vi "AudioStreamer.Close.vi"() -> (0 "success":bool)   [LabVIEW 2020]
panel:
  out "error out":errorcluster
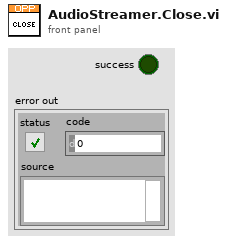
[diagram p1: front panel]
types:
  T1 = enum32{"Bad", "Idle", "Run top level", "Running"}
  T2 = enum32{"Invalid", "Standard", "Closed", "Hidden", "Minimized", "Maximized"}
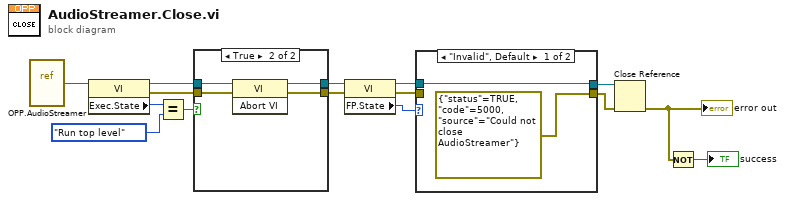
[diagram p0: block diagram]
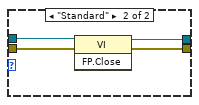
[diagram p2: hidden frame]
diagram:
  n1 = vi-ref "OPP.AudioStreamer.vi"() -> (w12:refnum<vi>)
  n2 = property class="VI"(reference=w12) -> (reference out=w15:refnum<vi>, error out=w14:errorcluster, "Exec.State"=w11:T1)  [unwired: 1 in]
  n3 = Equal?(x=w11, y=T1."Run top level" ("Execution:State")) -> (x = y?=w10:bool)
  n4 = case shown="True" w10 {
    tunnel: w15 -> [w17 w21]
    tunnel: w14 -> [w16 w20]
    tunnel: [w17 w19] -> w7
    tunnel: [w16 w18] -> w6
    frame False {
    }
    frame True {
      n5 = invoke class="VI" method="Abort VI"(reference=w21, error in=w20) -> (reference out=w19:refnum<vi>, error out=w18:errorcluster)  [unwired: 1 in, 1 out]
    }
  }
  n6 = property class="VI"(reference=w7, error in=w6) -> (reference out=w5:refnum<vi>, error out=w1:errorcluster, "FP.State"=w4:T2)
  n7 = case shown="\"Invalid\", Default" w4 {
    tunnel: [w22 w27] -> w3
    tunnel: [errorcluster {"status"=TRUE, "code"=5000, "source"="Could not close AudioStreamer"} ("error out") w26] -> w2
    tunnel: w5 -> [w22 w25]
    tunnel: w1 -> [_ w24]
    frame "Invalid", Default {
    }
    frame "Standard" {
      n8 = invoke class="VI" method="FP.Close"(reference=w25, error in=w24) -> (reference out=w27:refnum<vi>, error out=w26:errorcluster)  [unwired: 1 in, 1 out]
    }
  }
  n9 = Close Reference(reference=w3, error in (no error)=w2) -> (error out=w8:errorcluster)
  "error out" <- w8
  n10 = Not(x=w8) -> (.not. x?=→"success":bool)
